vi "Set Dummy Data.vi"(8 "error in (no error)":errorcluster, 10 "Dummy Data":T1, 11 "LogicIO in":refnum<class "LogicIO.lvclass">) -> (0 "error out":errorcluster, 3 "LogicIO out":refnum<class "LogicIO.lvclass">)   [LabVIEW 2016, in "Hardware.lvlib" / "LogicIO.lvlib" / "LogicIO.lvclass"]
uses:
  <userlib>/Common Components/Hardware/LogicIO/LogicIO/LogicIO.lvclass
  <userlib>/Common Components/Hardware/LogicIO/LogicIO/Dummy Data.ctl
  <userlib>/Common Components/Hardware/Abstract System/VacuumLine/VacuumLine/Valve Complex.ctl
  <userlib>/Common Components/Hardware/Abstract System/VacuumLine/VacuumLine/Logic Cluster.ctl
  <userlib>/Common Components/Hardware/Abstract System/VacuumLine/VacuumLine/VacuumLine.lvclass
panel:
  # "Pin#"
  # "Location"
  # "Tolerance"
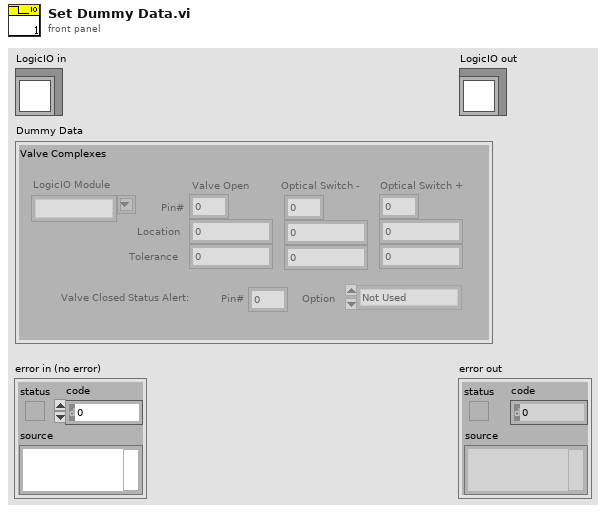
[diagram p1: front panel]
types:
  T1 = typedef "Hardware.lvlib/LogicIO.lvlib/LogicIO.lvclass/Dummy Data.ctl" = cluster{"Valve Complexes":T2[]}
  T2 = typedef "Hardware.lvlib/VacuumLine.lvlib/VacuumLine.lvclass/Valve Complex.ctl" = cluster{"LogicIO Module":string, "Valve Open":T3, "Optical Switch -":T3, "Optical Switch +":T3, "Valve Closed Status Alert":cluster{"Pin#":u8, "Option":enum16{"Not Used", "Normally Closed"}}}
  T3 = typedef "Hardware.lvlib/VacuumLine.lvlib/VacuumLine.lvclass/Logic Cluster.ctl" = cluster{"Pin#":u8, "Location":dbl, "Tolerance":dbl}
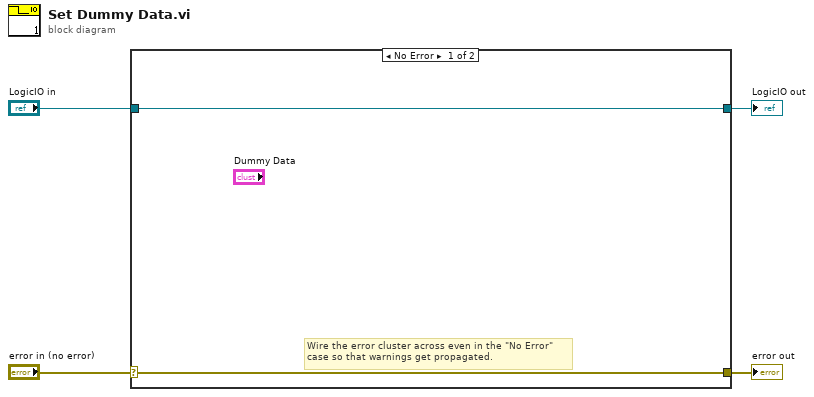
[diagram p0: block diagram]
diagram:
  n1 = case shown="No Error" "error in (no error)" {
    selector: "error in (no error)" -> [w5 w8]
    tunnel: [w5 w8] -> w3
    tunnel: [w6 w7] -> w1
    tunnel: "LogicIO in" -> [w6 w7]
    frame No Error {
      # "Wire the error cluster across even in the \"No Error\"\ncase so that warnings get propagated."
    }
    frame Error {
    }
  }
  "error out" <- w3
  "LogicIO out" <- w1
